vi "Example 1553 Initialization.vi"   [LabVIEW 2016]
uses:
  1553 SubComponent/1553 SubComponent.lvclass
  Utilities/FPGA Interface/FPGA Interface.lvclass
  1553 Component/1553 Component.lvclass
  Remote Terminal/Remote Terminal.lvclass
  Bus Monitor/Bus Monitor.lvclass
  Bus Controller/Bus Controller.lvclass
  1553 Board/1553 Board.lvclass
  D:/SVN/Products/BCI-1553/Software/Development/2016/RealTime/1553 SubComponent/1553 SubComponent.lvclass
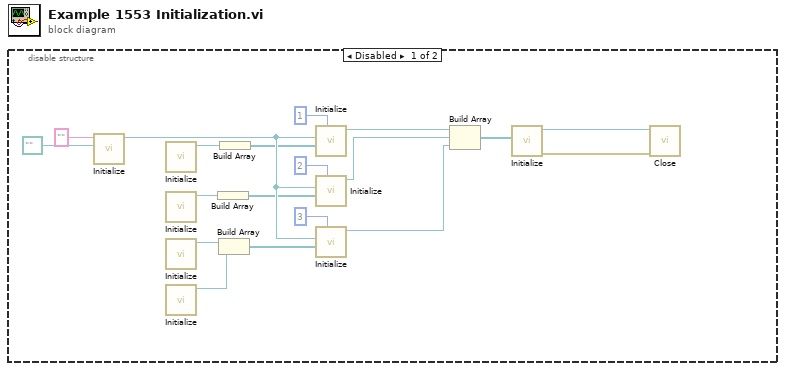
[diagram p0: block diagram]
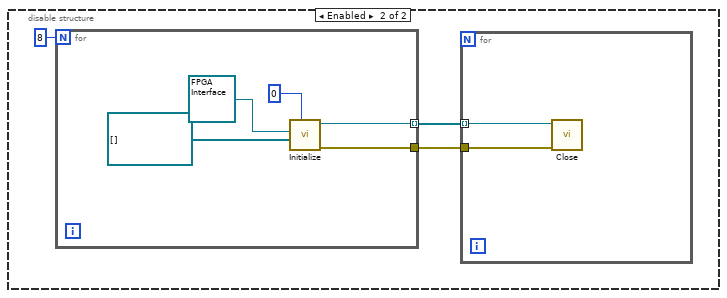
[diagram p2: hidden frame]
diagram:
  n1 = disable-structure shown="Disabled" {
    frame Disabled {
      n2 = call "Initialize.vi"("Bitfile path"=path "", "Device address"="") -> ("FPGA Interface out"=w19:refnum<class "FPGA Interface.lvclass">)  [unwired: 8 in, 1 out]
      n3 = call "Initialize.vi"() -> ("Bus Monitor out"=w12:refnum<class "Bus Monitor.lvclass">)  [unwired: 10 in, 1 out]
      n4 = call "Initialize.vi"() -> ("Bus Controller out"=w14:refnum<class "Bus Controller.lvclass">)  [unwired: 10 in, 1 out]
      n5 = call "Initialize.vi"() -> ("Remote Terminal out"=w17:refnum<class "Remote Terminal.lvclass">)  [unwired: 10 in, 1 out]
      n6 = call "Initialize.vi"() -> ("Remote Terminal out"=w18:refnum<class "Remote Terminal.lvclass">)  [unwired: 10 in, 1 out]
      n7 = Build Array(w14) -> (w13:refnum<class "Bus Controller.lvclass">[])
      n8 = Build Array(w17, w18) -> (w16:refnum<class "Remote Terminal.lvclass">[])
      n9 = Build Array(w12) -> (w11:refnum<class "Bus Monitor.lvclass">[])
      n10 = call "Initialize.vi"("Component ID (1-8)"=u8 1 ("Component ID"), "SubComponents"=w11, "FPGA Interface"=w19) -> ("1553 Component out"=w6:refnum<class "1553 Component.lvclass">)  [unwired: 7 in, 1 out]
      n11 = call "Initialize.vi"("Component ID (1-8)"=u8 2 ("Component ID"), "SubComponents"=w13, "FPGA Interface"=w19) -> ("1553 Component out"=w5:refnum<class "1553 Component.lvclass">)  [unwired: 7 in, 1 out]
      n12 = call "Initialize.vi"("Component ID (1-8)"=u8 3 ("Component ID"), "SubComponents"=w16, "FPGA Interface"=w19) -> ("1553 Component out"=w4:refnum<class "1553 Component.lvclass">)  [unwired: 7 in, 1 out]
      n13 = Build Array(w6, w5, w4) -> (w3:refnum<class "1553 Component.lvclass">[])
      n14 = call "Initialize.vi"("Components"=w3) -> ("error out"=w1:errorcluster, "1553 Board out"=w2:refnum<class "1553 Board.lvclass">)  [unwired: 9 in]
      n15 = call-dynamic "Close.vi"("error in (no error)"=w1, "1553 Board in"=w2) -> ()  [unwired: 9 in, 1 out]
    }
    frame Enabled {
      n16 = for {
        N: 8 -> [_]
        tunnel: [w29] -> w22 mode=indexing
        tunnel: [w28] -> w21
        n17 = call "Initialize.vi"("Component ID (1-8)"=u8 0 ("Component ID"), "SubComponents"=refnum<class "1553 SubComponent.lvclass">[] [], "FPGA Interface"=refnum<class "FPGA Interface.lvclass"> refnum) -> ("error out"=w28:errorcluster, "1553 Component out"=w29:refnum<class "1553 Component.lvclass">)  [unwired: 7 in]
      }
      n18 = for {
        tunnel: w22 -> [w24] mode=indexing
        tunnel: w21 -> [w23]
        n19 = call-dynamic "Close.vi"("error in (no error)"=w23, "1553 Component in"=w24) -> ()  [unwired: 9 in, 1 out]
      }
    }
  }
